vi "Convert Encoder to Distance (Feet).vi"(10 "Right Encoder":dbl, 11 "Left Encoder":dbl) -> (2 "Right Encoder":dbl, 3 "Left Distance":dbl)   [LabVIEW 2016]
doc: "Converts encoder reading to distance in feet; NEEDS TO BE IMPLEMENTED"
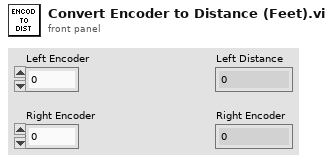
[diagram p1: front panel]
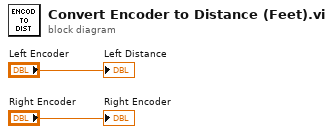
[diagram p0: block diagram]
diagram:
  "Left Distance" <- "Left Encoder"
  "Right Encoder" <- "Right Encoder"
